vi "finish.vi"(11 "ActiveSuspension.lvclass":refnum<class "Qube.lvclass">) -> (0 "error out":errorcluster)   [LabVIEW 2020, in "Qube.lvclass"]
uses:
  Qube.lvclass
  Qube.lvclass/Qube.ctl
  <vilib>/Quanser/Rapid Control Prototyping Toolkit/hardware/HIL Board/HIL Close.vi
  <vilib>/Quanser/Rapid Control Prototyping Toolkit/hardware/HIL Board/HIL Board.lvclass
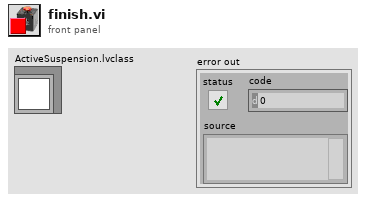
[diagram p1: front panel]
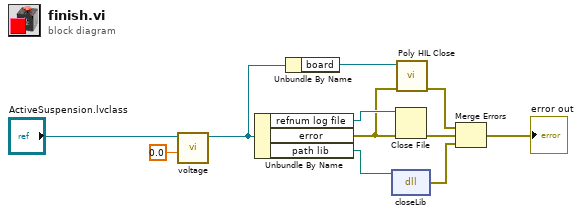
[diagram p0: block diagram]
diagram:
  n1 = call "voltage.vi"("u"=0.0, "Qube"="ActiveSuspension.lvclass") -> ("Qube"=w9:refnum<class "Qube.lvclass">)  [unwired: 9 in]
  n2 = Unbundle By Name(w9) -> ("refnum log file"=w11:refnum<file>, "error"=w3:errorcluster, "path lib"=w6:path)
  n3 = Unbundle By Name(w9) -> ("board"=w8:refnum<class "HIL Board.lvclass">)
  n4 = dll-call lib="Users/philippe/Desktop/cpp/LibLoader/libLoader.so" fn="closeLib"(path in=w6) -> (error out=w1:errorcluster)  [unwired: 3 in, 1 out]
  n5 = Close File(refnum=w11, error in=w3) -> (error out=w7:errorcluster)  [unwired: 1 out]
  n6 = call-poly <vilib>:"Poly HIL Close.vi"("error in (no error)"=w3, "board in"=w8) -> ("error out"=w2:errorcluster)  [unwired: 9 in]
  n7 = Merge Errors(w2, w7, w1) -> (→"error out":errorcluster)
